vi "SerialBusHound - 複製.vi"() -> ()   [LabVIEW 2011]
uses:
  Variable/gSTOP.vi
panel:
  out "status":bool
  in  "VISA-RS232":refnum<visa-resource-name>="COM5"
  in  "VISA-USB":refnum<visa-resource-name>
  in  "stop bits":u16(ring)=10 items=["1.0"=10, "1.5"=15, "2.0"=20]
  in  "parity":u16
  in  "data bits":u16=8 min=5 max=8 step=1
  in  "baud rate":u32=115200
  in  "Com Port":bool
  in  "USB":bool
  in  "IN 2":bool=TRUE
  in  "OUT 2":bool=TRUE
  in  "Broadcast":bool
  in  "Unicast":bool
  in  "OUT Packet":u8[](array[numeric])=[84, 49, 1, 42, 73, 68, 78, 63, 0, 0, 0, 0, 0, 0, 0, 0] format="%02x"
  out "IN     Packet":u8[](array[numeric])=[84, 49, 1, 42, 73, 68, 78, 63, 0, 0, 0, 0, 0, 0, 0, 0] format="%02x"
  out "String":string="Serial Bus Hound User Guilde.\n1. Push RUN Buttom To Execution.\r\n2. Push Clear Buttom To Clear Data Scream.\n\nAuthor by Ares."
  in  "ms":u32=100
  in  "Capacity":i32=16
  in  "Max":i32=500
  in  "clear":bool
  in  "run":bool
  out "Progress Bar":i32(slide)=432 scale=-1.0..1000000.0
  out "status":string="Running"
  # "BASIC"
  # "VISA - COM"
  # "VISA - USB"
  # "Phase"
  # "Data"
  # "Desccription"
  # "Settings"
  # "Capture Capacity"
  # "bytes"
  # "Rate"
  # "Max Record Length"
  # "bytes"
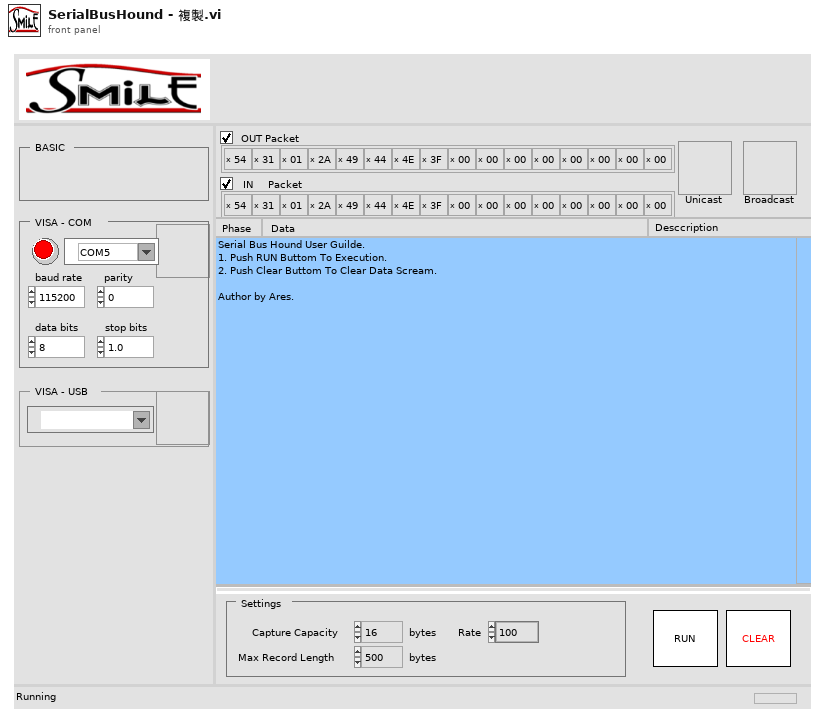
[diagram p1: front panel]
types:
  T1 = cluster{"VISA-RS232":refnum<visa-resource-name>, "baud rate":u32, "data bits":u16, "parity":u16, "stop bits":u16}
  T2 = enum16{"Open", "R", "W", "R->W", "W->R", "Close"}
  T3 = enum16{"Loopback", "*IDN?", "Unicast", "Broadcast"}
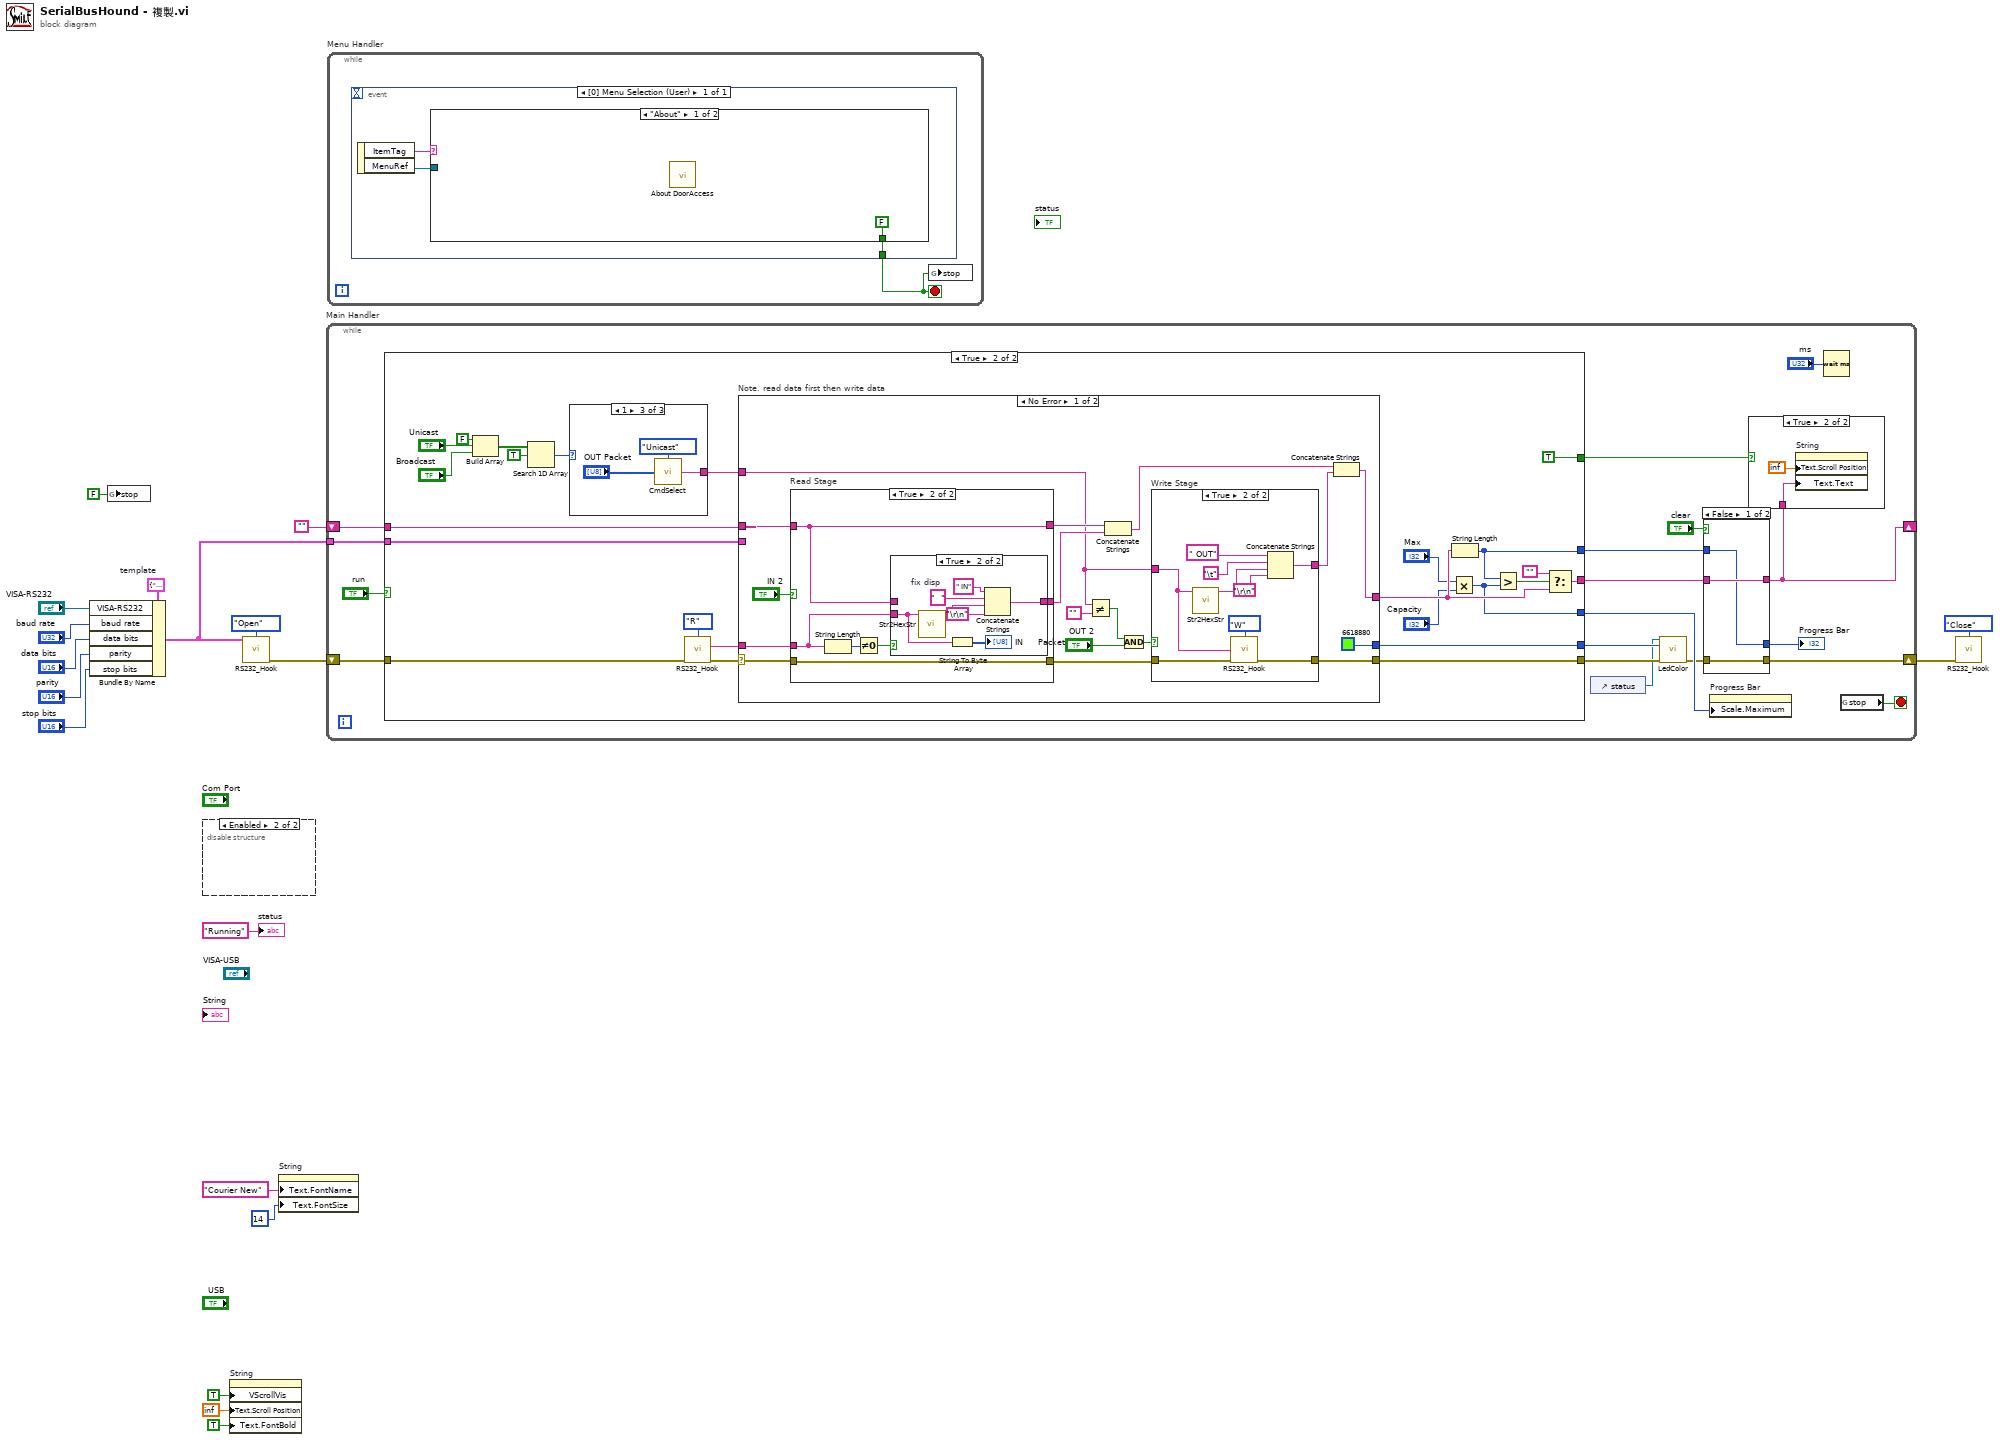
[diagram p0: block diagram]
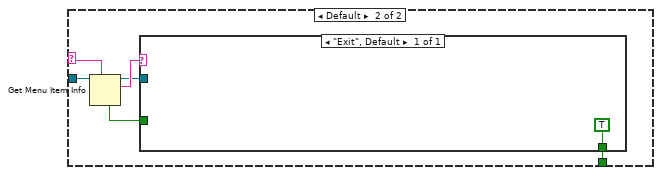
[diagram p2: hidden frame]
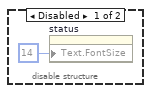
[diagram p3: hidden frame]
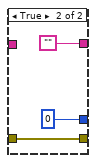
[diagram p5: hidden frame]
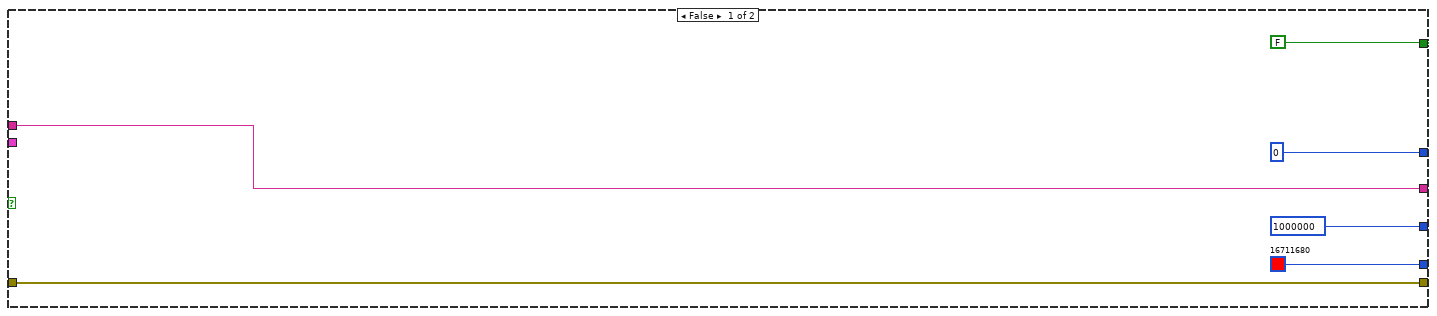
[diagram p6: hidden frame]
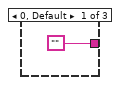
[diagram p7: hidden frame]
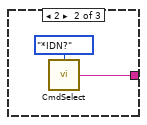
[diagram p8: hidden frame]
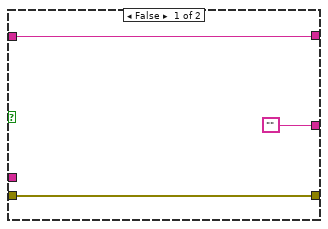
[diagram p9: hidden frame]
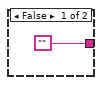
[diagram p10: hidden frame]
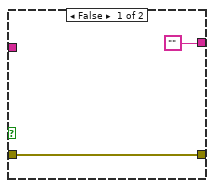
[diagram p11: hidden frame]
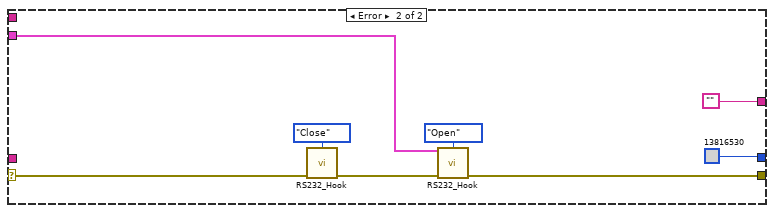
[diagram p12: hidden frame]
diagram:
  w8 = T1 {"VISA-RS232"="", "baud rate"=0, "data bits"=0, "parity"=0, "stop bits"=0}  # template
  n1 = Bundle By Name(cluster=w8, "VISA-RS232"="VISA-RS232", "baud rate"="baud rate", "data bits"="data bits", "parity"="parity", "stop bits"="stop bits") -> (w2:T1)
  n2 = global write "gSTOP.vi" "stop"(FALSE ("stop")) -> ()
  n3 = disable-structure shown="Enabled" {
    frame Disabled {
      n4 = property on="status" class="Str"("Text.FontSize"=u32 14 ("Text.Font:Size")) -> ()  [unwired: 2 in, 2 out]
    }
    frame Enabled {
    }
  }
  n5 = property on="String" class="Str"("VScrollVis"=TRUE ("Vertical Scrollbar Visible"), "Text.Scroll Position"=inf, "Text.FontBold"=TRUE ("Text.Font:Bold")) -> ()  [unwired: 2 in, 2 out]
  n6 = call "RS232_Hook.vi"("RS232 Config"=w2, "Mode"=T2."Open") -> ("error out"=w18:errorcluster)  [unwired: 12 in, 1 out]
  n7 = property on="String" class="Str"("Text.FontName"="Courier New" ("Text.Font:Name"), "Text.FontSize"=u32 14 ("Text.Font:Size")) -> ()  [unwired: 2 in, 2 out]
  n8 = while "Main Handler" {
    shift-right: [w29] -> w16
    shift-left: w18 -> [w37]
    tunnel: w2 -> [w36]
    shift-right: [w27] -> _
    shift-left: "" -> [w35]
    stop <- w34 stop-if-true
    n9 = case shown="True" "run" {
      tunnel: w37 -> [w52 w76]
      tunnel: [w52 w54] -> w24
      tunnel: w36 -> [_ w74]
      tunnel: w35 -> [w50 w73]
      tunnel: [0 w69] -> w32
      tunnel: [1000000 w68] -> w26
      tunnel: [w50 w67] -> w31
      tunnel: [FALSE TRUE] -> w25
      tunnel: [u32 16711680 w53] -> w22
      frame False {
      }
      frame True {
        n10 = Build Array(FALSE ("element"), "Unicast", "Broadcast") -> (w60:bool[])
        n11 = Search 1D Array(1D array=w60, element=TRUE) -> (index of element=w57:i32)  [unwired: 1 in]
        n12 = case shown="1" w57 {
          tunnel: ["" w78 w81] -> w56
          frame 0, Default {
          }
          frame 2 {
            n13 = call "CmdSelect.vi"("Cmd"=T3."*IDN?") -> ("string"=w78:string)  [unwired: 14 in]
          }
          frame 1 {
            n14 = call "CmdSelect.vi"("Cmd"=T3."Unicast", "Array"="OUT Packet") -> ("string"=w81:string)  [unwired: 13 in]
          }
        }
        n15 = call "RS232_Hook.vi"("Mode"=T2."R", "error in"=w76) -> ("data out"=w72:string, "error out"=w75:errorcluster)  [unwired: 12 in]
        n16 = case "Note. read data first then write data" shown="No Error" w75 {
          selector: w75 -> [w98 w133]
          tunnel: [w95 w131] -> w54
          tunnel: w74 -> [_ w130]
          tunnel: w73 -> [w94 _]
          tunnel: [w87 ""] -> w70
          tunnel: w72 -> [w96 _]
          tunnel: w56 -> [w85 _]
          tunnel: [u32 6618880 u32 13816530] -> w53
          frame No Error {
            n17 = case "Read Stage" shown="True" "IN 2" {
              tunnel: ["" w104] -> w93
              tunnel: w94 -> [w100 w103]
              tunnel: w98 -> [w102 w105]
              tunnel: [w102 w105] -> w97
              tunnel: w96 -> [_ w106]
              tunnel: [w100 w103] -> w92
              frame False {
              }
              frame True {
                n18 = String Length(string=w106) -> (length=w108:i32)
                n19 = Not Equal To 0?(x=w108) -> (x != 0?=w107:bool)
                n20 = case shown="True" w107 {
                  tunnel: ["" w114] -> w104
                  tunnel: w106 -> [_ w110]
                  tunnel: w103 -> [_ _]
                  frame False {
                  }
                  frame True {
                    w113 = "  "  # fix disp
                    n21 = call "Str2HexStr.vi"("data out"=w110) -> ("String"=w115:string)  [unwired: 10 in]
                    n22 = String To Byte Array(string=w110) -> (unsigned byte array=→"IN     Packet":u8[])
                    n23 = Concatenate Strings(" IN" ("string"), w113, w115, "\r\n") -> (w114:string)
                  }
                }
              }
            }
            n24 = Not Equal?(x=w85, y="") -> (x != y?=w84:bool)
            n25 = Concatenate Strings(w92, w93) -> (w91:string)
            n26 = And(x=w84, y="OUT 2") -> (x .and. y?=w89:bool)
            n27 = case "Write Stage" shown="True" w89 {
              tunnel: ["" w124] -> w90
              tunnel: w97 -> [w118 w121]
              tunnel: [w118 w120] -> w95
              tunnel: w85 -> [_ w119]
              frame False {
              }
              frame True {
                n28 = call "Str2HexStr.vi"("data out"=w119) -> ("String"=w125:string)  [unwired: 10 in]
                n29 = call "RS232_Hook.vi"("Mode"=T2."W", "data in"=w119, "error in"=w121) -> ("error out"=w120:errorcluster)  [unwired: 11 in, 1 out]
                n30 = Concatenate Strings(" OUT" ("string"), "\t", w125, "\r\n") -> (w124:string)
              }
            }
            n31 = Concatenate Strings(w91, w90) -> (w87:string)
          }
          frame Error {
            n32 = call "RS232_Hook.vi"("Mode"=T2."Close", "error in"=w133) -> ("error out"=w132:errorcluster)  [unwired: 12 in, 1 out]
            n33 = call "RS232_Hook.vi"("RS232 Config"=w130, "Mode"=T2."Open", "error in"=w132) -> ("error out"=w131:errorcluster)  [unwired: 11 in, 1 out]
          }
        }
        n34 = Multiply(x="Max", y="Capacity") -> (x*y=w68:i32)
        n35 = String Length(string=w70) -> (length=w69:i32)
        n36 = Greater?(x=w69, y=w68) -> (0:w66:bool)
        n37 = Select(t="", s=w66, f=w70) -> (s? t:f=w67:string)
      }
    }
    n38 = control-ref of="status"() -> (w21:refnum<vi>)
    n39 = call "LedColor.vi"("Boolean in"=w21, "Color Box"=w22, "error in (no error)"=w24) -> ("error out"=w23:errorcluster)  [unwired: 12 in]
    n40 = case shown="False" "clear" {
      tunnel: w32 -> [w42 _]
      tunnel: w31 -> [w43 _]
      tunnel: [w42 0] -> w30
      tunnel: [w43 ""] -> w27
      tunnel: w23 -> [w41 w45]
      tunnel: [w41 w45] -> w29
      frame False {
      }
      frame True {
      }
    }
    "Progress Bar" <- w30
    n41 = property on="Progress Bar" class="Slide (strict)"("Scale.Maximum"=w26) -> ()  [unwired: 2 in, 2 out]
    n42 = case shown="True" w25 {
      tunnel: w27 -> [_ w39]
      frame False {
      }
      frame True {
        n43 = property on="String" class="Str"("Text.Scroll Position"=inf, "Text.Text"=w39) -> ()  [unwired: 2 in, 2 out]
      }
    }
    n44 = Wait (ms)(milliseconds to wait="ms") -> ()  [unwired: 1 out]
    n45 = global read "gSTOP.vi" "stop"() -> (w34:bool)
  }
  n46 = while "Menu Handler" {
    stop <- w136 stop-if-true
    n47 = event shown="[0] Menu Selection (User)" {
      selector: _ -> [_]
      dyn-events: _ -> [_]
      timeout: _ -> [_]
      tunnel: [w137] -> w136
      event Menu Selection (User) {
        n48 = event-data() -> ("ItemTag"=w138:string, "MenuRef"=w139:refnum<k9>)  [unwired: 1 in]
        n49 = case shown="\"About\"" w138 {
          selector: w138 -> [_ w145]
          tunnel: w139 -> [_ w146]
          tunnel: [FALSE w143] -> w137
          frame "About" {
            n50 = call "About DoorAccess.vi"() -> ()  [unwired: 1 in]
          }
          frame Default {
            n51 = Get Menu Item Info(7:w145, 11:w146) -> (2:w144:string, 3:w142:refnum<k9>, 4:w141:bool)  [unwired: 1 in, 4 out]
            n52 = case shown="\"Exit\", Default" w144 {
              tunnel: [TRUE] -> w143
              tunnel: w142 -> [_]
              tunnel: w141 -> [_]
              frame "Exit", Default {
              }
            }
          }
        }
      }
    }
    n53 = global write "gSTOP.vi" "stop"(w136) -> ()
  }
  n54 = call "RS232_Hook.vi"("Mode"=T2."Close", "error in"=w16) -> ()  [unwired: 12 in, 2 out]
  "status" <- "Running" ("String 2")
